vi "Blue to yellow 1.vi"   [LabVIEW 2019]
uses:
  Global Var.vi
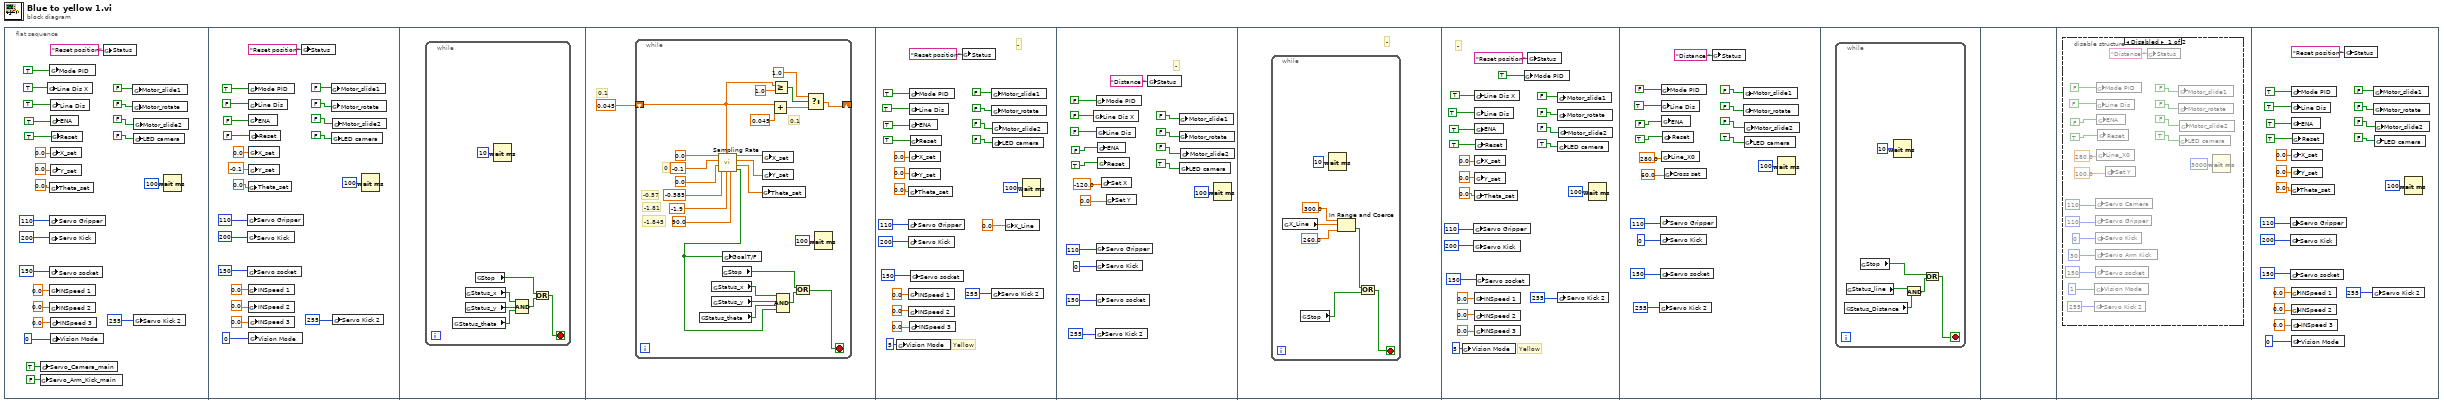
[diagram p0: block diagram]
diagram:
  n1 = flat-sequence {
    frame #0 {
      n2 = global write "Global Var.vi" "Servo_Arm_Kick_main"(FALSE ("Mode PID")) -> ()
      n3 = global write "Global Var.vi" "Servo_Camera_main"(TRUE ("Mode PID")) -> ()
      n4 = global write "Global Var.vi" "Line Dis X"(TRUE ("Mode PID")) -> ()
      n5 = global write "Global Var.vi" "Servo Gripper"(u8 110 ("Servo Camera")) -> ()
      n6 = global write "Global Var.vi" "Servo Kick"(u8 200 ("Servo Camera")) -> ()
      n7 = global write "Global Var.vi" "Servo socket"(u8 150 ("Servo Camera")) -> ()
      n8 = global write "Global Var.vi" "Mode PID"(TRUE ("Mode PID")) -> ()
      n9 = global write "Global Var.vi" "Theta_set"(0.0 ("Theta_set")) -> ()
      n10 = global write "Global Var.vi" "INSpeed 1"(0.0 ("X_set")) -> ()
      n11 = global write "Global Var.vi" "INSpeed 2"(0.0 ("Y_set")) -> ()
      n12 = global write "Global Var.vi" "Line Dis"(TRUE ("Mode PID")) -> ()
      n13 = global write "Global Var.vi" "ENA"(TRUE ("ENA")) -> ()
      n14 = global write "Global Var.vi" "X_set"(0.0 ("X_set")) -> ()
      n15 = global write "Global Var.vi" "Y_set"(0.0 ("Y_set")) -> ()
      n16 = global write "Global Var.vi" "INSpeed 3"(0.0 ("Theta_set")) -> ()
      n17 = global write "Global Var.vi" "Vision Mode"(i16 0 ("Vision Mode")) -> ()
      n18 = global write "Global Var.vi" "Reset"(TRUE ("ENA")) -> ()
      n19 = global write "Global Var.vi" "Status"("Reset position" ("Status")) -> ()
      n20 = global write "Global Var.vi" "Motor_slide1"(FALSE ("Mode PID")) -> ()
      n21 = global write "Global Var.vi" "Motor_rotate"(FALSE ("ENA")) -> ()
      n22 = global write "Global Var.vi" "LED camera"(FALSE ("LED camera")) -> ()
      n23 = global write "Global Var.vi" "Motor_slide2"(FALSE ("ENA")) -> ()
      n24 = global write "Global Var.vi" "Servo Kick 2"(u8 255 ("Servo Camera")) -> ()
      n25 = Wait (ms)(milliseconds to wait=u32 100) -> ()  [unwired: 1 out]
    }
    frame #1 {
      n26 = global write "Global Var.vi" "Servo Gripper"(u8 110 ("Servo Camera")) -> ()
      n27 = global write "Global Var.vi" "Servo Kick"(u8 200 ("Servo Camera")) -> ()
      n28 = global write "Global Var.vi" "Servo socket"(u8 150 ("Servo Camera")) -> ()
      n29 = global write "Global Var.vi" "Theta_set"(0.0 ("Theta_set")) -> ()
      n30 = global write "Global Var.vi" "INSpeed 1"(0.0 ("X_set")) -> ()
      n31 = global write "Global Var.vi" "INSpeed 2"(0.0 ("Y_set")) -> ()
      n32 = global write "Global Var.vi" "Mode PID"(TRUE ("Mode PID")) -> ()
      n33 = global write "Global Var.vi" "Line Dis"(FALSE ("Mode PID")) -> ()
      n34 = global write "Global Var.vi" "ENA"(FALSE ("ENA")) -> ()
      n35 = global write "Global Var.vi" "X_set"(0.0 ("X_set")) -> ()
      n36 = global write "Global Var.vi" "Y_set"(-0.1 ("Y_set")) -> ()
      n37 = global write "Global Var.vi" "INSpeed 3"(0.0 ("Theta_set")) -> ()
      n38 = global write "Global Var.vi" "Vision Mode"(i16 0 ("Vision Mode")) -> ()
      n39 = global write "Global Var.vi" "Reset"(FALSE ("ENA")) -> ()
      n40 = global write "Global Var.vi" "Status"("Reset position" ("Status")) -> ()
      n41 = global write "Global Var.vi" "Motor_slide1"(FALSE ("Mode PID")) -> ()
      n42 = global write "Global Var.vi" "Motor_rotate"(FALSE ("ENA")) -> ()
      n43 = global write "Global Var.vi" "LED camera"(FALSE ("LED camera")) -> ()
      n44 = global write "Global Var.vi" "Motor_slide2"(FALSE ("ENA")) -> ()
      n45 = global write "Global Var.vi" "Servo Kick 2"(u8 255 ("Servo Camera")) -> ()
      n46 = Wait (ms)(milliseconds to wait=u32 100) -> ()  [unwired: 1 out]
    }
    frame #2 {
      n47 = while {
        stop <- w48 stop-if-true
        n48 = global read "Global Var.vi" "Status_theta"() -> (w50:bool)
        n49 = global read "Global Var.vi" "Status_x"() -> (w51:bool)
        n50 = global read "Global Var.vi" "Status_y"() -> (w52:bool)
        n51 = global read "Global Var.vi" "Stop"() -> (w46:bool)
        n52 = Wait (ms)(milliseconds to wait=u32 10) -> ()  [unwired: 1 out]
        n53 = Compound Arithmetic op=AND(w51, w52, w50) -> (w47:bool)
        n54 = Or(x=w46, y=w47) -> (x .or. y?=w48:bool)
      }
    }
    frame #3 {
      # "0.1"
      n55 = while {
        shift-right: [w56] -> _
        shift-left: 0.045 -> [w54]
        stop <- w73 stop-if-true
        # "-1.845"
        # "0"
        # "0.1"
        # "-1.81"
        # "-0.57"
        n56 = global read "Global Var.vi" "Status_theta"() -> (w75:bool)
        n57 = global read "Global Var.vi" "Status_x"() -> (w76:bool)
        n58 = global read "Global Var.vi" "Status_y"() -> (w77:bool)
        n59 = call "Sampling Rate.vi"("input a1"=90.0, "input y1"=-1.9, "T(0-1)"=w54, "input x1"=-0.585, "input a0"=0.0, "input y0"=-0.1, "input x0"=0.0) -> ("GoalT/F"=w61:bool, "a_output"=w68:dbl, "y_output"=w69:dbl, "x_output"=w70:dbl)  [unwired: 1 in]
        n60 = global read "Global Var.vi" "Stop"() -> (w71:bool)
        n61 = global write "Global Var.vi" "GoalT/F"(w61) -> ()
        n62 = global write "Global Var.vi" "Theta_set"(w68) -> ()
        n63 = global write "Global Var.vi" "X_set"(w70) -> ()
        n64 = global write "Global Var.vi" "Y_set"(w69) -> ()
        n65 = Add(x=w54, y=0.045) -> (x+y=w59:dbl)
        n66 = Greater Or Equal?(x=w54, y=1.0) -> (x >= y?=w58:bool)
        n67 = Compound Arithmetic op=AND(w76, w77, w75, w61) -> (w72:bool)
        n68 = Or(x=w71, y=w72) -> (x .or. y?=w73:bool)
        n69 = Select(t=1.0, s=w58, f=w59) -> (s? t:f=w56:dbl)
        n70 = Wait (ms)(milliseconds to wait=u32 100) -> ()  [unwired: 1 out]
      }
    }
    frame #4 {
      # "-"
      # "Yellow"
      n71 = global write "Global Var.vi" "Vision Mode"(i16 5 ("Vision Mode")) -> ()
      n72 = global write "Global Var.vi" "Servo Gripper"(u8 110 ("Servo Camera")) -> ()
      n73 = global write "Global Var.vi" "Servo Kick"(u8 200 ("Servo Camera")) -> ()
      n74 = global write "Global Var.vi" "Theta_set"(0.0 ("Theta_set")) -> ()
      n75 = global write "Global Var.vi" "INSpeed 1"(0.0 ("X_set")) -> ()
      n76 = global write "Global Var.vi" "INSpeed 2"(0.0 ("Y_set")) -> ()
      n77 = global write "Global Var.vi" "Mode PID"(TRUE ("Mode PID")) -> ()
      n78 = global write "Global Var.vi" "Line Dis"(TRUE ("Mode PID")) -> ()
      n79 = global write "Global Var.vi" "ENA"(TRUE ("ENA")) -> ()
      n80 = global write "Global Var.vi" "X_set"(0.0 ("X_set")) -> ()
      n81 = global write "Global Var.vi" "Y_set"(0.0 ("Y_set")) -> ()
      n82 = global write "Global Var.vi" "INSpeed 3"(0.0 ("Theta_set")) -> ()
      n83 = global write "Global Var.vi" "Reset"(TRUE ("ENA")) -> ()
      n84 = global write "Global Var.vi" "Servo socket"(u8 150 ("Servo Camera")) -> ()
      n85 = global write "Global Var.vi" "Status"("Reset position" ("Status")) -> ()
      n86 = global write "Global Var.vi" "Motor_slide1"(FALSE ("Mode PID")) -> ()
      n87 = global write "Global Var.vi" "Motor_rotate"(FALSE ("ENA")) -> ()
      n88 = global write "Global Var.vi" "Servo Kick 2"(u8 255 ("Servo Camera")) -> ()
      n89 = global write "Global Var.vi" "LED camera"(FALSE ("LED camera")) -> ()
      n90 = global write "Global Var.vi" "Motor_slide2"(FALSE ("ENA")) -> ()
      n91 = global write "Global Var.vi" "X_Line"(0.0 ("X_set")) -> ()
      n92 = Wait (ms)(milliseconds to wait=u32 100) -> ()  [unwired: 1 out]
    }
    frame #5 {
      # "-"
      n93 = global write "Global Var.vi" "Line Dis X"(FALSE ("Mode PID")) -> ()
      n94 = global write "Global Var.vi" "Servo Kick 2"(u8 255 ("Servo Camera")) -> ()
      n95 = global write "Global Var.vi" "Mode PID"(FALSE ("Mode PID")) -> ()
      n96 = global write "Global Var.vi" "Servo Gripper"(u8 110 ("Servo Camera")) -> ()
      n97 = global write "Global Var.vi" "Servo Kick"(u8 0 ("Servo Camera")) -> ()
      n98 = global write "Global Var.vi" "Servo socket"(u8 150 ("Servo Camera")) -> ()
      n99 = global write "Global Var.vi" "Line Dis"(FALSE ("Mode PID")) -> ()
      n100 = global write "Global Var.vi" "ENA"(FALSE ("ENA")) -> ()
      n101 = global write "Global Var.vi" "Reset"(TRUE ("ENA")) -> ()
      n102 = global write "Global Var.vi" "Set X"(-120.0 ("Y_set")) -> ()
      n103 = global write "Global Var.vi" "Set Y"(0.0 ("Y_set")) -> ()
      n104 = global write "Global Var.vi" "Status"("Distance " ("Status")) -> ()
      n105 = global write "Global Var.vi" "Motor_slide1"(FALSE ("Mode PID")) -> ()
      n106 = global write "Global Var.vi" "Motor_rotate"(FALSE ("ENA")) -> ()
      n107 = global write "Global Var.vi" "LED camera"(TRUE ("LED camera")) -> ()
      n108 = global write "Global Var.vi" "Motor_slide2"(FALSE ("ENA")) -> ()
      n109 = Wait (ms)(milliseconds to wait=u32 100) -> ()  [unwired: 1 out]
    }
    frame #6 {
      # "-"
      n110 = while {
        stop <- w122 stop-if-true
        n111 = global read "Global Var.vi" "X_Line"() -> (w120:dbl)
        n112 = global read "Global Var.vi" "Stop"() -> (w121:bool)
        n113 = Wait (ms)(milliseconds to wait=u32 10) -> ()  [unwired: 1 out]
        n114 = In Range and Coerce(upper limit=300.0, x=w120, lower limit=260.0) -> (In Range?=w117:bool)  [unwired: 1 out]
        n115 = Or(x=w117, y=w121) -> (x .or. y?=w122:bool)
      }
    }
    frame #7 {
      # "-"
      # "Yellow"
      n116 = global write "Global Var.vi" "Vision Mode"(i16 5 ("Vision Mode")) -> ()
      n117 = global write "Global Var.vi" "Servo Gripper"(u8 110 ("Servo Camera")) -> ()
      n118 = global write "Global Var.vi" "Servo Kick"(u8 200 ("Servo Camera")) -> ()
      n119 = global write "Global Var.vi" "Line Dis X"(TRUE ("Mode PID")) -> ()
      n120 = global write "Global Var.vi" "Theta_set"(0.0 ("Theta_set")) -> ()
      n121 = global write "Global Var.vi" "INSpeed 1"(0.0 ("X_set")) -> ()
      n122 = global write "Global Var.vi" "INSpeed 2"(0.0 ("Y_set")) -> ()
      n123 = global write "Global Var.vi" "Line Dis"(TRUE ("Mode PID")) -> ()
      n124 = global write "Global Var.vi" "ENA"(TRUE ("ENA")) -> ()
      n125 = global write "Global Var.vi" "X_set"(0.0 ("X_set")) -> ()
      n126 = global write "Global Var.vi" "Y_set"(0.0 ("Y_set")) -> ()
      n127 = global write "Global Var.vi" "INSpeed 3"(0.0 ("Theta_set")) -> ()
      n128 = global write "Global Var.vi" "Reset"(TRUE ("ENA")) -> ()
      n129 = global write "Global Var.vi" "Servo socket"(u8 150 ("Servo Camera")) -> ()
      n130 = global write "Global Var.vi" "Mode PID"(TRUE ("Mode PID")) -> ()
      n131 = global write "Global Var.vi" "Status"("Reset position" ("Status")) -> ()
      n132 = global write "Global Var.vi" "Motor_slide1"(FALSE ("Mode PID")) -> ()
      n133 = global write "Global Var.vi" "Motor_rotate"(FALSE ("ENA")) -> ()
      n134 = global write "Global Var.vi" "Servo Kick 2"(u8 255 ("Servo Camera")) -> ()
      n135 = global write "Global Var.vi" "LED camera"(TRUE ("LED camera")) -> ()
      n136 = global write "Global Var.vi" "Motor_slide2"(FALSE ("ENA")) -> ()
      n137 = Wait (ms)(milliseconds to wait=u32 100) -> ()  [unwired: 1 out]
    }
    frame #8 {
      n138 = global write "Global Var.vi" "Servo Kick 2"(u8 255 ("Servo Camera")) -> ()
      n139 = global write "Global Var.vi" "Servo Gripper"(u8 110 ("Servo Camera")) -> ()
      n140 = global write "Global Var.vi" "Servo Kick"(u8 0 ("Servo Camera")) -> ()
      n141 = global write "Global Var.vi" "Servo socket"(u8 150 ("Servo Camera")) -> ()
      n142 = global write "Global Var.vi" "Mode PID"(FALSE ("Mode PID")) -> ()
      n143 = global write "Global Var.vi" "Line Dis"(TRUE ("Mode PID")) -> ()
      n144 = global write "Global Var.vi" "ENA"(FALSE ("ENA")) -> ()
      n145 = global write "Global Var.vi" "Line_X0"(280.0 ("Y_set")) -> ()
      n146 = global write "Global Var.vi" "Reset"(TRUE ("ENA")) -> ()
      n147 = global write "Global Var.vi" "Cross set"(60.0 ("Y_set")) -> ()
      n148 = global write "Global Var.vi" "Status"("Distance " ("Status")) -> ()
      n149 = global write "Global Var.vi" "Motor_slide1"(FALSE ("Mode PID")) -> ()
      n150 = global write "Global Var.vi" "Motor_rotate"(FALSE ("ENA")) -> ()
      n151 = global write "Global Var.vi" "LED camera"(TRUE ("LED camera")) -> ()
      n152 = global write "Global Var.vi" "Motor_slide2"(FALSE ("ENA")) -> ()
      n153 = Wait (ms)(milliseconds to wait=u32 100) -> ()  [unwired: 1 out]
    }
    frame #9 {
      n154 = while {
        stop <- w166 stop-if-true
        n155 = global read "Global Var.vi" "Status_Distance"() -> (w162:bool)
        n156 = global read "Global Var.vi" "Status_line"() -> (w163:bool)
        n157 = global read "Global Var.vi" "Stop"() -> (w165:bool)
        n158 = Wait (ms)(milliseconds to wait=u32 10) -> ()  [unwired: 1 out]
        n159 = And(x=w163, y=w162) -> (x .and. y?=w164:bool)
        n160 = Or(x=w165, y=w164) -> (x .or. y?=w166:bool)
      }
    }
    frame #10 {
    }
    frame #11 {
      n161 = disable-structure shown="Disabled" {
        frame Disabled {
          n162 = global write "Global Var.vi" "Servo Kick 2"(u8 255 ("Servo Camera")) -> ()
          n163 = global write "Global Var.vi" "Vision Mode"(i16 1 ("Vision Mode")) -> ()
          n164 = global write "Global Var.vi" "Servo Camera"(u8 110 ("Servo Camera")) -> ()
          n165 = global write "Global Var.vi" "Servo Gripper"(u8 110 ("Servo Camera")) -> ()
          n166 = global write "Global Var.vi" "Servo Kick"(u8 0 ("Servo Camera")) -> ()
          n167 = global write "Global Var.vi" "Servo Arm Kick"(u8 30 ("Servo Camera")) -> ()
          n168 = global write "Global Var.vi" "Servo socket"(u8 150 ("Servo Camera")) -> ()
          n169 = global write "Global Var.vi" "Mode PID"(FALSE ("Mode PID")) -> ()
          n170 = global write "Global Var.vi" "Line Dis"(FALSE ("Mode PID")) -> ()
          n171 = global write "Global Var.vi" "ENA"(FALSE ("ENA")) -> ()
          n172 = global write "Global Var.vi" "Line_X0"(280.0 ("Y_set")) -> ()
          n173 = global write "Global Var.vi" "Reset"(TRUE ("ENA")) -> ()
          n174 = global write "Global Var.vi" "Set Y"(100.0 ("Y_set")) -> ()
          n175 = global write "Global Var.vi" "Status"("Distance " ("Status")) -> ()
          n176 = global write "Global Var.vi" "Motor_slide1"(FALSE ("Mode PID")) -> ()
          n177 = global write "Global Var.vi" "Motor_rotate"(FALSE ("ENA")) -> ()
          n178 = global write "Global Var.vi" "LED camera"(TRUE ("LED camera")) -> ()
          n179 = global write "Global Var.vi" "Motor_slide2"(FALSE ("ENA")) -> ()
          n180 = Wait (ms)(milliseconds to wait=u32 3000) -> ()  [unwired: 1 out]
        }
        frame Enabled {
        }
      }
    }
    frame #12 {
      n181 = global write "Global Var.vi" "Servo Gripper"(u8 110 ("Servo Camera")) -> ()
      n182 = global write "Global Var.vi" "Servo Kick"(u8 200 ("Servo Camera")) -> ()
      n183 = global write "Global Var.vi" "Servo socket"(u8 150 ("Servo Camera")) -> ()
      n184 = global write "Global Var.vi" "Theta_set"(0.0 ("Theta_set")) -> ()
      n185 = global write "Global Var.vi" "INSpeed 1"(0.0 ("X_set")) -> ()
      n186 = global write "Global Var.vi" "INSpeed 2"(0.0 ("Y_set")) -> ()
      n187 = global write "Global Var.vi" "Mode PID"(TRUE ("Mode PID")) -> ()
      n188 = global write "Global Var.vi" "Line Dis"(TRUE ("Mode PID")) -> ()
      n189 = global write "Global Var.vi" "ENA"(TRUE ("ENA")) -> ()
      n190 = global write "Global Var.vi" "X_set"(0.0 ("X_set")) -> ()
      n191 = global write "Global Var.vi" "Y_set"(0.0 ("Y_set")) -> ()
      n192 = global write "Global Var.vi" "INSpeed 3"(0.0 ("Theta_set")) -> ()
      n193 = global write "Global Var.vi" "Vision Mode"(i16 0 ("Vision Mode")) -> ()
      n194 = global write "Global Var.vi" "Reset"(TRUE ("ENA")) -> ()
      n195 = global write "Global Var.vi" "Status"("Reset position" ("Status")) -> ()
      n196 = global write "Global Var.vi" "Servo Kick 2"(u8 255 ("Servo Camera")) -> ()
      n197 = global write "Global Var.vi" "Motor_slide1"(FALSE ("Mode PID")) -> ()
      n198 = global write "Global Var.vi" "Motor_rotate"(FALSE ("ENA")) -> ()
      n199 = global write "Global Var.vi" "LED camera"(FALSE ("LED camera")) -> ()
      n200 = global write "Global Var.vi" "Motor_slide2"(FALSE ("ENA")) -> ()
      n201 = Wait (ms)(milliseconds to wait=u32 100) -> ()  [unwired: 1 out]
    }
  }
